vi "Demo.vi"() -> ()   [LabVIEW 2013]
uses:
  <vilib>/Utility/miscctls.llb/LV3DPointTypeDef.ctl
  <vilib>/picture/3D Picture Control/NI_3D Picture Control.lvlib
panel:
  in  "stop":bool
  in  "Right Pos":dbl(slide) scale=-4.0..10.0
  in  "Left Pos":dbl(slide) scale=-4.0..10.0
  out "3D Picture":refnum<vi>(3d-picture)
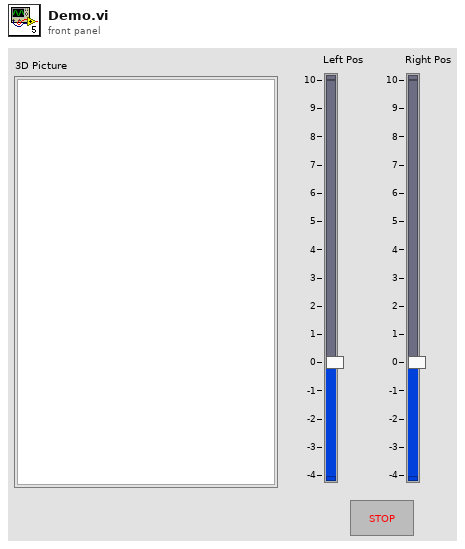
[diagram p1: front panel]
types:
  T1 = typedef "LV3DPointTypeDef.ctl" = cluster{"X":sgl, "Y":sgl, "Z":sgl}
  T2 = typedef "BIRD-3D.ctl" = cluster{"BIRD Object":refnum<vi>, "Left Pedal":refnum<vi>, "Right Pedal":refnum<vi>}
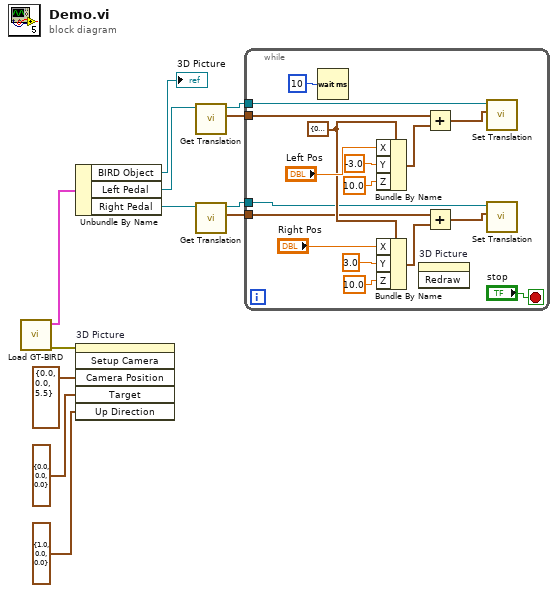
[diagram p0: block diagram]
diagram:
  n1 = call "Load GT-BIRD.vi"() -> ("error out"=w1:errorcluster, "BIRD-3D output"=w12:T2)  [unwired: 10 in]
  n2 = Unbundle By Name(w12) -> ("BIRD Object"=→"3D Picture":refnum<vi>, "Left Pedal"=w11:refnum<vi>, "Right Pedal"=w8:refnum<vi>)
  n3 = invoke on="3D Picture" class="SceneGraphDisp (strict)" method="Setup Camera"(error in=w1, "Camera Position"=T1 {"X"=0.0, "Y"=0.0, "Z"=5.5}, "Target"=T1 {"X"=0.0, "Y"=0.0, "Z"=0.0}, "Up Direction"=T1 {"X"=1.0, "Y"=0.0, "Z"=0.0}) -> ()  [unwired: 2 in, 6 out]
  n4 = call <vilib>:"Get Translation.vi"("Scene Object"=w11) -> ("Transformation:Get Translation"=w9:cluster{"X":sgl, "Y":sgl, "Z":sgl}, "Scene Object"=w10:refnum<vi>)  [unwired: 8 in, 1 out]
  n5 = call <vilib>:"Get Translation.vi"("Scene Object"=w8) -> ("Transformation:Get Translation"=w6:cluster{"X":sgl, "Y":sgl, "Z":sgl}, "Scene Object"=w7:refnum<vi>)  [unwired: 8 in, 1 out]
  n6 = while {
    tunnel: w10 -> [w28]
    tunnel: w9 -> [w27]
    tunnel: w7 -> [w21]
    tunnel: w6 -> [w22]
    stop <- "stop" stop-if-true
    w24 = cluster{"X":sgl, "Y":sgl, "Z":sgl} {"X"=0.0, "Y"=0.0, "Z"=0.0} ("y")
    n7 = Wait (ms)(milliseconds to wait=u32 10) -> ()  [unwired: 1 out]
    n8 = Bundle By Name(cluster=w24, "X"="Left Pos", "Y"=sgl -3.0, "Z"=sgl 10.0) -> (w25:cluster{"X":sgl, "Y":sgl, "Z":sgl})
    n9 = Bundle By Name(cluster=w24, "X"="Right Pos", "Y"=sgl 3.0, "Z"=sgl 10.0) -> (w20:cluster{"X":sgl, "Y":sgl, "Z":sgl})
    n10 = invoke on="3D Picture" class="SceneGraphDisp (strict)" method="Redraw"() -> ()  [unwired: 3 in, 3 out]
    n11 = Add(x=w27, y=w25) -> (x+y=w18:cluster{"X":sgl, "Y":sgl, "Z":sgl})
    n12 = Add(x=w22, y=w20) -> (x+y=w19:cluster{"X":sgl, "Y":sgl, "Z":sgl})
    n13 = call <vilib>:"Set Translation.vi"("Translation"=w18, "Scene Object"=w28) -> ()  [unwired: 8 in, 2 out]
    n14 = call <vilib>:"Set Translation.vi"("Translation"=w19, "Scene Object"=w21) -> ()  [unwired: 8 in, 2 out]
  }
